vi "Set Stage Max Velocity.vi"(8 "error in":errorcluster, 10 "Max Velocity":dbl, 11 ".NET Refnum in":refnum<k24>) -> (0 "error out":errorcluster, 3 ".NET Refnum out":refnum<k24>)   [LabVIEW 2020, in "ThorlabsLTS.lvclass"]
uses:
  ThorlabsLTS.lvclass
  C:/GEECS/Developers Version/source/Device Drivers/ThorLabsLTS/Thorlabs.MotionControl.IntegratedStepperMotorsCLI.dll
  Thorlabs.MotionControl.IntegratedStepperMotorsCLI.dll
  C:/GEECS/Developers Version/source/Device Drivers/ThorLabsLTS/Thorlabs.MotionControl.GenericMotorCLI.dll
  Thorlabs.MotionControl.GenericMotorCLI.dll
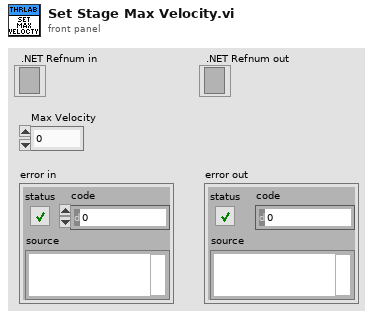
[diagram p1: front panel]
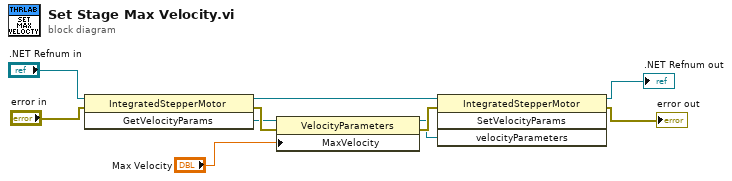
[diagram p0: block diagram]
diagram:
  n1 = invoke class="IntegratedStepperMotor" method="GetVelocityParams"(reference=".NET Refnum in", error in="error in") -> (reference out=w8:refnum<k24>, error out=w4:errorcluster, "GetVelocityParams"=w3:refnum<k24>)  [unwired: 1 in]
  n2 = property class="VelocityParameters"(reference=w3, error in=w4, "MaxVelocity"="Max Velocity") -> (reference out=w6:refnum<k24>, error out=w7:errorcluster)
  n3 = invoke class="IntegratedStepperMotor" method="SetVelocityParams"(reference=w8, error in=w7, "velocityParameters"=w6) -> (reference out=→".NET Refnum out":refnum<k24>, error out=→"error out":errorcluster)  [unwired: 1 in, 2 out]
